vi "OAT Polar Calc Scale Specs.vi"(1 "desired font(Application)":T4(ring)=enum."Application Font", 2 "scale definition":T1={"coordinate 1"=5, "value 1"=5.0, "coordinate 2"=5, "value 2"=5.0, "log"=FALSE, "fmt and prec"={"format"=enum."Hex", "precision"=0}} {"value 2" format="%.2f"; "value 1" format="%.2f"}, 3 "scale attributes":T2={"horizontal"=TRUE, "left/top"=FALSE, "draw bar"=FALSE, "line color"=0, "text color"=0}, 5 "[user-specified font]":T3) -> (7 "scale specs":cluster{"coordinate":i16, "label":string}[](array[cluster])=[{"coordinate"=7, "label"="1"}, {"coordinate"=23, "label"="2"}])   [LabVIEW 2017]
doc: "Takes a specification for a Cartesian style scale and calculates the coordinates and labels to use for the scale."
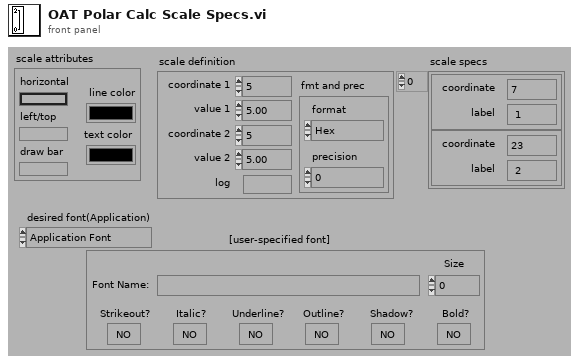
[diagram p1: front panel]
types:
  T1 = cluster{"coordinate 1":i16, "value 1":dbl, "coordinate 2":i16, "value 2":dbl, "log":bool, "fmt and prec":cluster{"format":enum8{"Decimal", "Scientific", "Engineering", "Binary", "Octal", "Hex"}, "precision":u8}}
  T2 = cluster{"horizontal":bool, "left/top":bool, "draw bar":bool, "line color":u32, "text color":u32}
  T3 = cluster{"Font Name:":string, "Size":i16, "Strikeout?":bool, "Italic?":bool, "Underline?":bool, "Outline?":bool, "Shadow?":bool, "Bold?":bool}
  T4 = enum16{"User-specified Font", "Application Font", "System Font", "Dialog Font"}
  T5 = cluster{"format":enum8{"Decimal", "Scientific", "Engineering", "Binary", "Octal", "Hex"}, "precision":u8}
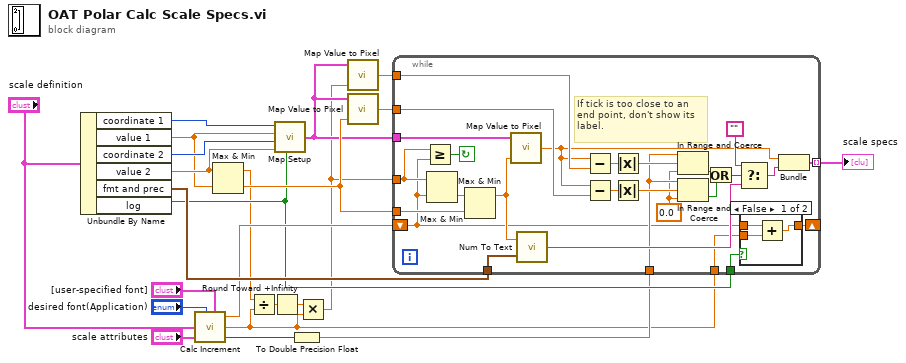
[diagram p0: block diagram]
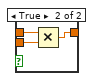
[diagram p2: hidden frame]
diagram:
  n1 = Unbundle By Name("scale definition") -> ("coordinate 1"=w18:i16, "value 1"=w1:dbl, "coordinate 2"=w21:i16, "value 2"=w2:dbl, "fmt and prec"=w22:T5, "log"=w9:bool)
  n2 = call <vilib>:"Calc Increment.vi"("desired font(Application)"="desired font(Application)", "scale definition"="scale definition", "scale attributes"="scale attributes", "[user-specified font]"="[user-specified font]") -> ("start"=w11:dbl, "increment"=w4:dbl, "text size"=w20:i16)  [unwired: 3 in]
  n3 = Max & Min(x=w2, y=w1) -> (max(x,y)=w6:dbl, min(x,y)=w19:dbl)
  n4 = Divide(x=w6, y=w4) -> (x/y=w7:dbl)
  n5 = Round Toward +Infinity(x=w7) -> (ceil(x): smallest int >= x=w5:dbl)
  n6 = call <vilib>:"Map Setup.vi"("coordinate 1"=w18, "value 1"=w1, "coordinate 2"=w21, "value 2"=w2, "log?(F)"=w9) -> ("scale factors"=w17:cluster{"a":dbl, "b":dbl, "log?(F)":bool})
  n7 = To Double Precision Float(number=w20) -> (double precision float=w8:dbl)
  n8 = Multiply(x=w5, y=w4) -> (x*y=w3:dbl)
  n9 = call <vilib>:"Map Value to Pixel.vi"("x"=w3, "scale factors"=w17) -> ("pixel"=w16:dbl)  [unwired: 1 in]
  n10 = call <vilib>:"Map Value to Pixel.vi"("x"=w19, "scale factors"=w17) -> ("pixel"=w15:dbl)  [unwired: 1 in]
  n11 = while {
    tunnel: w9 -> [w24]
    tunnel: w15 -> [w34]
    tunnel: w16 -> [w42]
    tunnel: w8 -> [w33]
    tunnel: w22 -> [w45]
    tunnel: [w49] -> w10 mode=indexing
    tunnel: w4 -> [w27]
    tunnel: w17 -> [w44]
    tunnel: w19 -> [w47]
    tunnel: w3 -> [w46]
    shift-left: w11 -> [w26]
    shift-right: [w25] -> _
    stop <- w48 continue-if-true
    w32 = 0.0
    # "If tick is too close to an\nend point, don't show its\nlabel."
    n12 = Greater Or Equal?(x=w46, y=w26) -> (x >= y?=w48:bool)
    n13 = Max & Min(x=w46, y=w26) -> (min(x,y)=w50:dbl)  [unwired: 1 out]
    n14 = Max & Min(x=w50, y=w47) -> (max(x,y)=w43:dbl)  [unwired: 1 out]
    n15 = call <vilib>:"Map Value to Pixel.vi"("x"=w43, "scale factors"=w44) -> ("pixel"=w28:dbl)  [unwired: 1 in]
    n16 = call <vilib>:"Num To Text.vi"("fmt and prec"=w45, "number"=w43) -> ("numeric string"=w38:string)
    n17 = Subtract(x=w28, y=w42) -> (x-y=w41:dbl)
    n18 = Subtract(x=w28, y=w34) -> (x-y=w35:dbl)
    n19 = Absolute Value(x=w41) -> (abs(x)=w40:dbl)
    n20 = Absolute Value(x=w35) -> (abs(x)=w36:dbl)
    n21 = In Range and Coerce(upper limit=w33, x=w40, lower limit=w32) -> (In Range?=w30:bool)  [unwired: 1 out]
    n22 = In Range and Coerce(upper limit=w33, x=w36, lower limit=w32) -> (In Range?=w29:bool)  [unwired: 1 out]
    n23 = Or(x=w30, y=w29) -> (x .or. y?=w31:bool)
    n24 = Select(t="", s=w31, f=w38) -> (s? t:f=w37:string)
    n25 = case shown="False" w24 {
      tunnel: w27 -> [w52 w56]
      tunnel: w26 -> [w51 w55]
      tunnel: [w53 w54] -> w25
      frame False {
        n26 = Add(x=w51, y=w52) -> (x+y=w53:dbl)
      }
      frame True {
        n27 = Multiply(x=w55, y=w56) -> (x*y=w54:dbl)
      }
    }
    n28 = Bundle("pixel"=w28, "numeric string"=w37) -> (w49:cluster{"pixel":dbl, "numeric string":string})  [unwired: 1 in]
  }
  "scale specs" <- w10
